vi "DataBase.Init.vi"(8 "error in (no error)":errorcluster, 11 "Path":path) -> (0 "error out":errorcluster, 3 "Refnum out":T1)   [LabVIEW 2019, in "Tools.lvlib"]
uses:
  <vilib>/addons/database/Connection.llb/Conn ObjectReference.ctl
  <vilib>/addons/database/Connection.llb/DB Tools Open Connec (Path).vi
  Tools.lvlib
  <vilib>/addons/database/NI_Database_API.lvlib
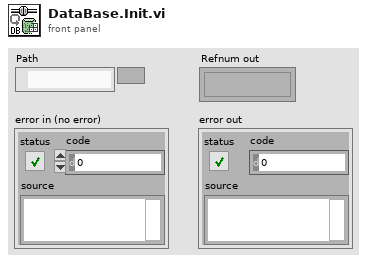
[diagram p1: front panel]
types:
  T1 = typedef "NI_Database_API.lvlib/Conn ObjectReference.ctl" = refnum<k1>
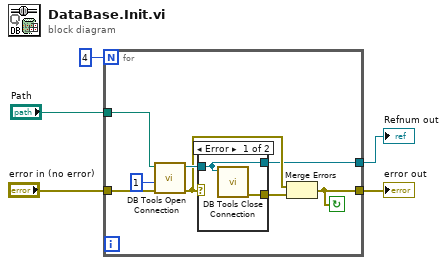
[diagram p0: block diagram]
diagram:
  n1 = for {
    N: 4 ("connection timeout (15)") -> [_]
    tunnel: [w7] -> w2
    tunnel: "Path" -> [w11]
    tunnel: "error in (no error)" -> [w12]
    tunnel: [w6] -> w1
    stop <- w6 continue-if-true
    n2 = call-poly <vilib>:"DB Tools Open Connection.vi"("error in (no error)"=w12, "connection timeout (15)"=1, "connection information"=w11) -> ("error out"=w9:errorcluster, "connection reference"=w10:T1)  [unwired: 5 in]
    n3 = case shown="Error" w9 {
      selector: w9 -> [_ w17]
      tunnel: w10 -> [w14 w16]
      tunnel: [w15 w17] -> w8
      tunnel: [w14 w16] -> w7
      frame Error {
        n4 = call <vilib>:"DB Tools Close Connection.vi"("connection reference"=w14) -> ("error out"=w15:errorcluster)  [unwired: 6 in]
      }
      frame No Error {
      }
    }
    n5 = Merge Errors(w9, w8) -> (w6:errorcluster)
  }
  "Refnum out" <- w2
  "error out" <- w1
